vi "imp_delay.vi"(1 "Meas":T1 {"Ud" format="%#.2f"; "P" format="%#.2f"; "Q" format="%#.2f"}, 2 "uc":cluster{"Pc":dbl, "Qc":dbl}) -> (0 "res-dt":dbl)   [LabVIEW 2021]
uses:
  General purpose/MEAS.ctl
panel:
  out "dQ":dbl
  out "dP":dbl
  out "dI_Q":dbl
  out "dI_P":dbl
  out "dt_Q":dbl
  out "dt_P":dbl
  in  "slew-rate [A/ms]":dbl=4.0 format="%#_13g"
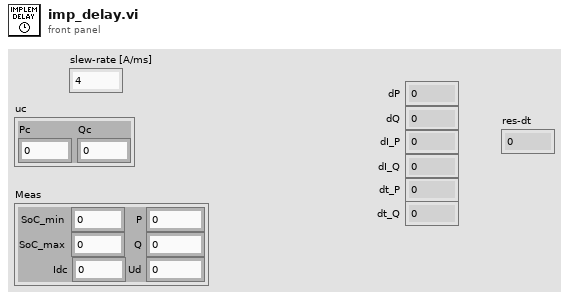
[diagram p1: front panel]
types:
  T1 = typedef "MEAS.ctl" = cluster{"P":dbl, "Q":dbl, "SoC_max":dbl, "SoC_min":dbl, "Ud":dbl, "Idc":dbl}
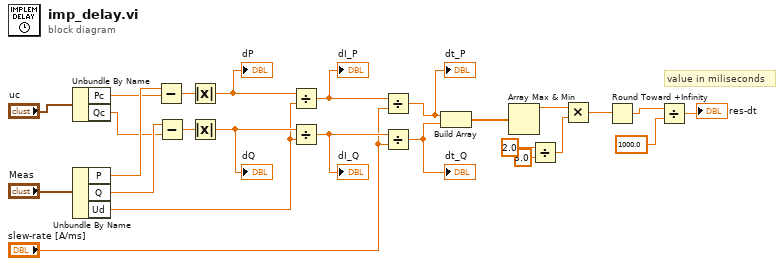
[diagram p0: block diagram]
diagram:
  # "value in miliseconds"
  n1 = Unbundle By Name("uc") -> ("Pc"=w7:dbl, "Qc"=w6:dbl)
  n2 = Unbundle By Name("Meas") -> ("P"=w25:dbl, "Q"=w24:dbl, "Ud"=w1:dbl)
  n3 = Subtract(x=w25, y=w7) -> (x-y=w23:dbl)
  n4 = Subtract(x=w24, y=w6) -> (x-y=w17:dbl)
  n5 = Absolute Value(x=w23) -> (abs(x)=w16:dbl)
  "dP" <- w16
  n6 = Absolute Value(x=w17) -> (abs(x)=w15:dbl)
  "dQ" <- w15
  n7 = Divide(x=w16, y=w1) -> (x/y=w22:dbl)
  "dI_P" <- w22
  n8 = Divide(x=w15, y=w1) -> (x/y=w21:dbl)
  "dI_Q" <- w21
  n9 = Divide(x=w22, y="slew-rate [A/ms]") -> (x/y=w14:dbl)
  "dt_P" <- w14
  n10 = Divide(x=w21, y="slew-rate [A/ms]") -> (x/y=w19:dbl)
  "dt_Q" <- w19
  n11 = Build Array(w14, w19) -> (w18:dbl[])
  n12 = Array Max & Min(array=w18) -> (max value=w12:dbl)  [unwired: 3 out]
  n13 = Divide(x=2.0, y=3.0) -> (x/y=w11:dbl)
  n14 = Multiply(x=w12, y=w11) -> (x*y=w13:dbl)
  n15 = Round Toward +Infinity(x=w13) -> (ceil(x): smallest int >= x=w4:dbl)
  n16 = Divide(x=w4, y=1000.0) -> (x/y=→"res-dt":dbl)
